vi "array_scaler.vi"(1 "array":dbl[](array[numeric]), 2 "scale":dbl) -> (9 "output array":dbl[](array[numeric]))   [LabVIEW 2014]
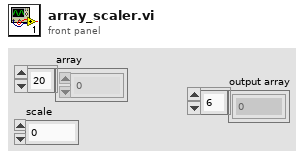
[diagram p1: front panel]
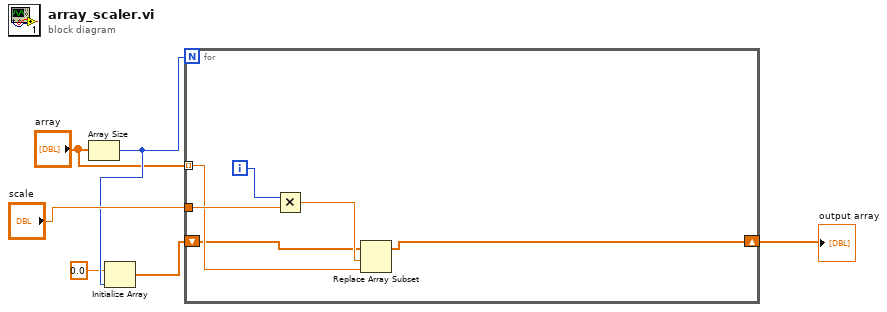
[diagram p0: block diagram]
diagram:
  n1 = Array Size(array="array") -> (size(s)=w5:i32)
  n2 = Initialize Array(0.0 ("element"), w5) -> (w2:dbl[])
  n3 = for {
    N: w5 -> [_]
    tunnel: "scale" -> [w12]
    tunnel: "array" -> [w9] mode=indexing
    shift-right: [w8] -> w1
    shift-left: w2 -> [w7]
    i -> [w11]
    n4 = Multiply(x=w11, y=w12) -> (x*y=w10:dbl)
    n5 = Replace Array Subset(array=w7, new element=w9, index=w10) -> (w8:dbl[])
  }
  "output array" <- w1
